vi "Simulated positioned arm.vi"(11 "Motor Type":T2=enum."775 pro") -> ()   [LabVIEW 2019]
uses:
  Motor Type.ctl
panel:
  out "2D Picture":picture
  in  "Type of motor control":enum32{"Manual", "PIDF"}(tab)
  in  "Effective Voltage":dbl[unit](slide) scale=-13.0..13.0
  in  "Setpoint":dbl(knob)
  out "Motor Position":dbl[unit] format="%#.2g"
  out "Motor position":dbl[unit](knob)
  out "Shaft Position":dbl[unit] format="%#.2g"
  out "Angular position":dbl[unit](knob)
  in  "Arm parameters":T1={"Mass at end"=1.0, "Length "=0.3, "Gear ratio (out/in)"=10.0, "Initial position"=0.0}
  in  "stop":bool
  in  "timestep":dbl[unit]=0.001 format="%#_3p"
  out "Motor Chart":cluster{"Free Speed":dbl, "Current":dbl[unit]}(graph)
  # "Restart VI if you change any\nof these values"
  # "Gravity"
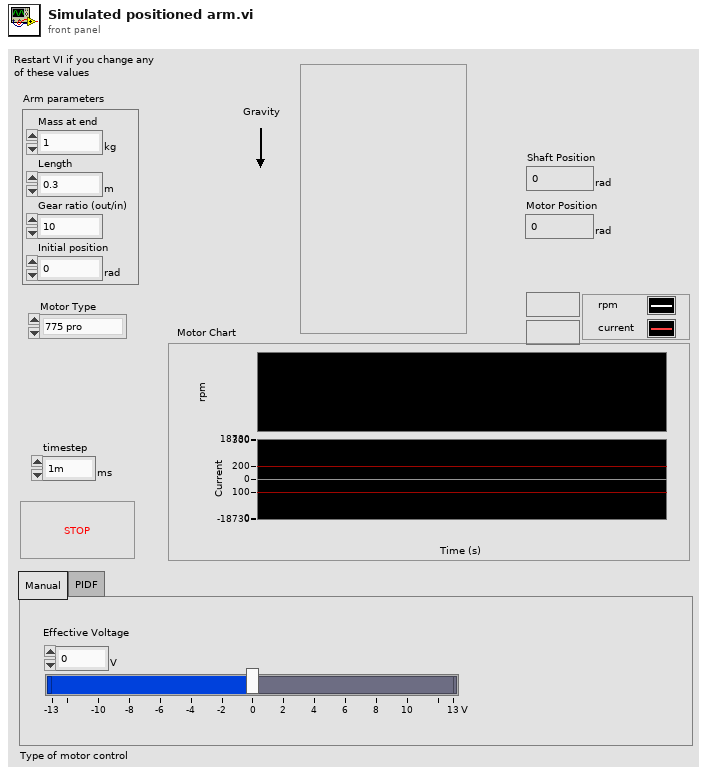
[diagram p1: front panel]
types:
  T1 = cluster{"Mass at end":dbl[unit], "Length ":dbl[unit], "Gear ratio (out/in)":dbl, "Initial position":dbl[unit]}
  T2 = typedef "Motor Type.ctl" = enum16{"Custom", "775 pro", "CIM", "miniCIM", "Neo", "Neo 550", "Falcon 500"}
  T3 = typedef "Motor Physical Values.ctl" = cluster{"Ratio (out/in)":dbl, "Moment of Inertia (kg m^2)":dbl[unit]}
  T4 = typedef "Motor Operating Values.ctl" = cluster{"Kv":dbl[unit], "R":dbl[unit], "Kt":dbl[unit], "Breaker Size":dbl[unit]}
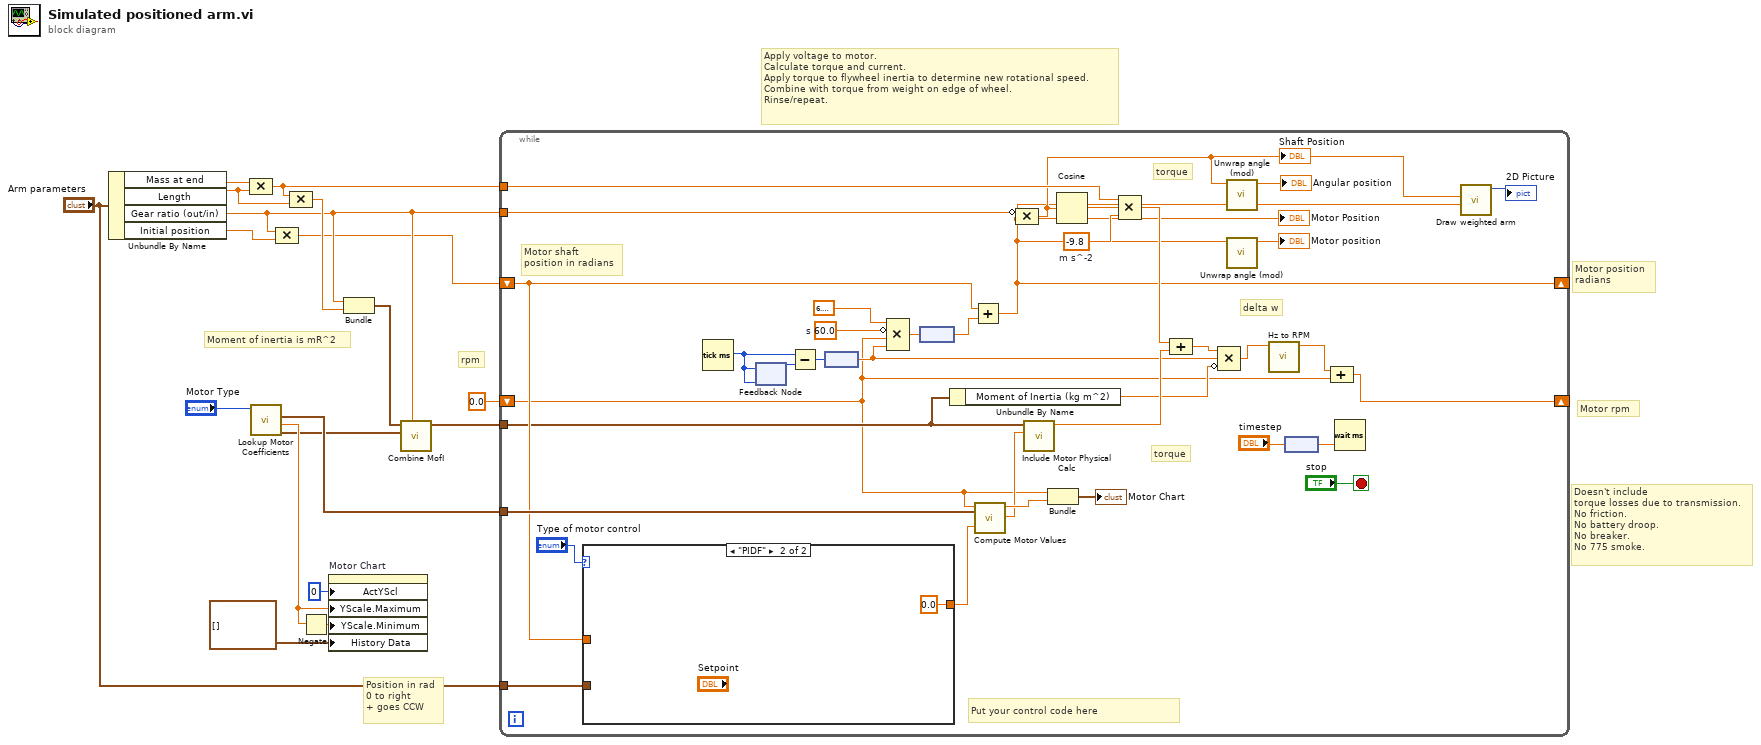
[diagram p0: block diagram]
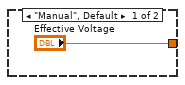
[diagram p2: hidden frame]
diagram:
  # "Doesn't include\ntorque losses due to transmission.\nNo friction.\nNo battery droop.\nNo breaker.\nNo 775 smoke."
  # "Position in rad\n0 to right\n+ goes CCW"
  # "Moment of inertia is mR^2"
  # "Motor position\nradians"
  # "rpm"
  # "Motor rpm"
  # "Apply voltage to motor.\nCalculate torque and current.\nApply torque to flywheel inertia to determine new rotational speed.\nCombine with torque from weight on edge of wheel.\nRinse/repeat."
  n1 = Unbundle By Name("Arm parameters") -> ("Mass at end"=w11:dbl[unit], "Length"=w9:dbl[unit], "Gear ratio (out/in)"=w3:dbl, "Initial position"=w4:dbl[unit])
  n2 = Compound Arithmetic op=MULTIPLY(w11, w9) -> (w10:dbl[unit])
  n3 = call "Lookup Motor Coefficients.vi"("Motor Type"="Motor Type") -> ("Physical Values"=w6:T3, "Free Speed"=w14:dbl, "Motor Model Values"=w13:T4)  [unwired: 7 in, 1 out]
  n4 = Compound Arithmetic op=MULTIPLY(w3, w4) -> (w2:dbl[unit])
  n5 = Compound Arithmetic op=MULTIPLY(w10, w9) -> (w8:dbl[unit])
  n6 = Negate(x=w14) -> (-x=w15:dbl)
  n7 = property on="Motor Chart" class="WFChart (strict)"("ActYScl"=0 ("Active Y Scale"), "YScale.Maximum"=w14, "YScale.Minimum"=w15, "History Data"=cluster{"Free Speed":dbl, "Current":dbl[unit]}[] []) -> ()  [unwired: 2 in, 2 out]
  n8 = Bundle("Gear ratio (out/in)"=w3, w8) -> (w7:cluster{"Gear ratio (out/in)":dbl, dbl[unit]})  [unwired: 1 in]
  n9 = call "Combine MofI.vi"("Final Ratio"=w3, "Rotational Mass 2"=w6, "Rotational Mass 1"=w7) -> ("Combined"=w5:T3)  [unwired: 8 in]
  n10 = while {
    tunnel: w13 -> [w55]
    shift-right: [w37] -> _
    shift-left: 0.0 -> [w23]
    tunnel: w5 -> [w29]
    shift-right: [w21] -> _
    shift-left: w2 -> [w33]
    tunnel: w3 -> [w38]
    tunnel: w10 -> [w39]
    tunnel: "Arm parameters" -> [w19]
    stop <- "stop" stop-if-true
    w26 = dbl[unit] -9.8  # m s^-2
    w44 = dbl[unit] 60.0  # s
    # "Put your control code here"
    # "torque"
    # "delta w"
    # "Motor shaft\nposition in radians"
    # "torque"
    n11 = case shown="\"PIDF\"" "Type of motor control" {
      tunnel: ["Effective Voltage" dbl[unit] 0.0 ("Effective Voltage")] -> w54
      tunnel: w33 -> [_ _]
      tunnel: w19 -> [_ _]
      frame "Manual", Default {
      }
      frame "PIDF" {
      }
    }
    n12 = Tick Count (ms)() -> (millisecond timer value=w50:u32)
    n13 = feedback-in #1(w50) -> ()
    n14 = feedback #1(w50) -> (w52:u32)
    n15 = Subtract(x=w50, y=w52) -> (x-y=w51:u32)
    n16 = node(w51) -> (w25:dbl[unit])
    n17 = Compound Arithmetic op=MULTIPLY(6.283185307179586, invert w44, w23, w25) -> (w42:dbl)
    n18 = node(w42) -> (w41:dbl[unit])
    n19 = Unbundle By Name(w29) -> ("Moment of Inertia (kg m^2)"=w24:dbl[unit])
    n20 = Add(x=w33, y=w41) -> (x+y=w21:dbl[unit])
    "Motor Position" <- w21
    n21 = call "Compute Motor Values.vi"("Effective Motor Voltage"=w54, "Motor Model Values"=w55, "motor speed (rpm)"=w23) -> ("Motor Torque"=w45:dbl[unit], "Current"=w49:dbl[unit])  [unwired: 6 in, 1 out]
    n22 = Compound Arithmetic op=MULTIPLY(invert w38, w21) -> (w22:dbl[unit])
    "Shaft Position" <- w22
    n23 = call "Include Motor Physical Calc.vi"("Motor Torque"=w45, "Physical Values"=w29) -> ("Flywheel Torque"=w32:dbl[unit])  [unwired: 8 in, 1 out]
    n24 = Bundle(w23, "Current"=w49) -> (→"Motor Chart":cluster{dbl, "Current":dbl[unit]})  [unwired: 1 in]
    n25 = Cosine(x=w22) -> (cos(x)=w40:dbl)
    n26 = Compound Arithmetic op=MULTIPLY(w39, w40, w26) -> (w31:dbl[unit])
    n27 = Compound Arithmetic op=ADD(w31, w32) -> (w30:dbl[unit])
    n28 = Compound Arithmetic op=MULTIPLY(w30, w25, invert w24) -> (w28:dbl[unit])
    n29 = call "Unwrap angle (mod).vi"("Numeric in"=w22) -> ("Numeric out"=→"Angular position":dbl[unit])  [unwired: 10 in]
    n30 = call "Unwrap angle (mod).vi"("Numeric in"=w21) -> ("Numeric out"=→"Motor position":dbl[unit])  [unwired: 10 in]
    n31 = call "Hz to RPM.vi"("Hz"=w28) -> ("speed out (rpm)"=w27:dbl)  [unwired: 10 in]
    n32 = node("timestep") -> (w46:dbl)
    n33 = Compound Arithmetic op=ADD(w27, w23) -> (w37:dbl)
    n34 = Wait (ms)(milliseconds to wait=w46) -> ()  [unwired: 1 out]
    n35 = call "Draw weighted arm.vi"("Motor Position"=w21, "Shaft Position"=w22) -> ("2D Picture"=→"2D Picture":picture)  [unwired: 9 in]
  }
